vi "snake and ladders.vi"() -> ()   [LabVIEW 2018]
panel:
  out "?":bool
  out "x":dbl
  out "Number":dbl
  in  "ROLL":bool
  in  "stop":bool
  out "Ring":u16(ring)
  # "98"
  # "93"
  # "94"
  # "97"
  # "95"
  # "100"
  # "91"
  # "92"
  # "99"
  # "96"
  # "87"
  # "85"
  # "90"
  # "89"
  # "82"
  # "84"
  # "88"
  # "86"
  # "83"
  # "81"
  # "80"
  # "74"
  # "78"
  # "72"
  # "75"
  # "76"
  # "77"
  # "79"
  # "71"
  # "73"
  # "61"
  # "62"
  # "67"
  # "68"
  # "69"
  # "64"
  # "66"
  # "65"
  # "70"
  # "63"
  # "57"
  # "52"
  # "53"
  # "58"
  # "54"
  # "55"
  # "56"
  # "59"
  # "51"
  # "60"
  # "45"
  # "46"
  # "47"
  # "43"
  # "42"
  # "48"
  # "49"
  # "50"
  # "41"
  # "44"
  # "31"
  # "33"
  # "35"
  # "37"
  # "32"
  # "36"
  # "39"
  # "34"
  # "40"
  # "38"
  # "27"
  # "26"
  # "30"
  # "22"
  # "23"
  # "24"
  # "29"
  # "21"
  # "25"
  # "28"
  # "15"
  # "17"
  # "11"
  # "12"
  # "19"
  # "20"
  # "14"
  # "16"
  # "13"
  # "18"
  # "8"
  # "7"
  # "3"
  # "2"
  # "4"
  # "5"
  # "9"
  # "10"
  # "6"
  # "1"
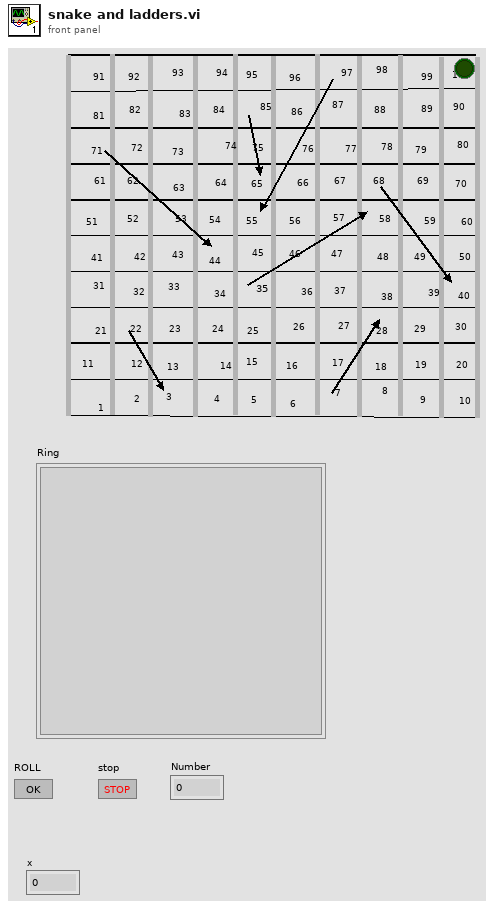
[diagram p1: front panel]
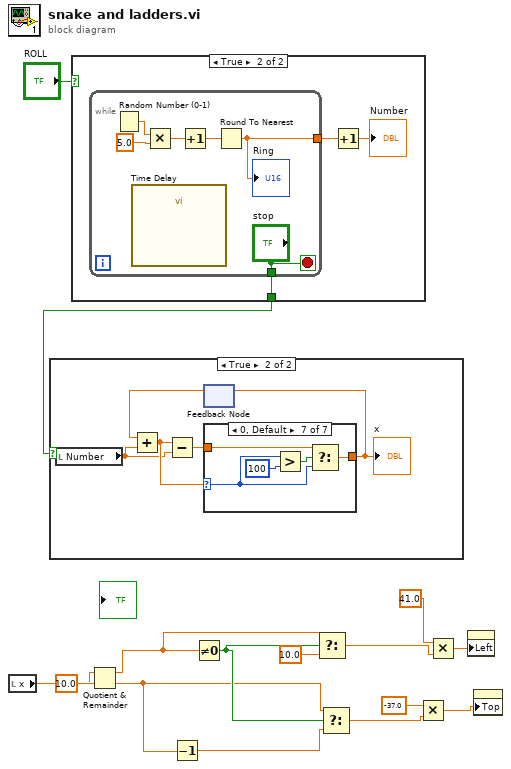
[diagram p0: block diagram]
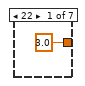
[diagram p3: hidden frame]
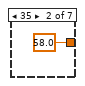
[diagram p4: hidden frame]
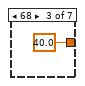
[diagram p5: hidden frame]
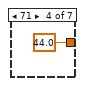
[diagram p6: hidden frame]
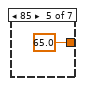
[diagram p7: hidden frame]
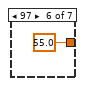
[diagram p8: hidden frame]
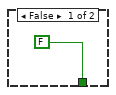
[diagram p9: hidden frame]
diagram:
  n1 = local read "x"() -> (w13:dbl)
  n2 = case shown="True" "ROLL" {
    tunnel: [FALSE ("Boolean") w17] -> w12
    frame False {
    }
    frame True {
      n3 = while {
        tunnel: [w21] -> w19
        tunnel: ["stop"] -> w17
        stop <- "stop" stop-if-true
        n4 = Random Number (0-1)() -> (number: 0 to 1=w25:dbl)
        n5 = call "Time Delay"() -> ()  [unwired: 11 in, 1 out]
        n6 = Multiply(x=w25, y=5.0) -> (x*y=w23:dbl)
        n7 = Increment(x=w23) -> (x+1=w22:dbl)
        n8 = Round To Nearest(number=w22) -> (nearest integer value=w21:dbl)
        "Ring" <- w21
      }
      n9 = Increment(x=w19) -> (x+1=→"Number":dbl)
    }
  }
  n10 = case shown="True" w12 {
    frame False {
    }
    frame True {
      n11 = local read "Number"() -> (w26:dbl)
      n12 = feedback #1() -> (w30:dbl)  [unwired: 1 in]
      n13 = Add(x=w30, y=w26) -> (x+y=w28:dbl)
      n14 = Subtract(x=w28, y=w26) -> (x-y=w27:dbl)
      n15 = case shown="0, Default" w28 {
        selector: w28 -> [_ _ _ _ _ _ w38]
        tunnel: [3.0 ("f") 58.0 ("f") 40.0 ("f") 44.0 ("f") 65.0 ("f") 55.0 ("f") w40] -> w29
        tunnel: w27 -> [_ _ _ _ _ _ w39]
        frame 22 {
        }
        frame 35 {
        }
        frame 68 {
        }
        frame 71 {
        }
        frame 85 {
        }
        frame 97 {
        }
        frame 0, Default {
          n16 = Greater?(x=w38, y=100 ("x")) -> (0:w41:bool)
          n17 = Select(t=w39, s=w41, f=w38) -> (s? t:f=w40:dbl)
        }
      }
      "x" <- w29
      n18 = feedback-in #1(w29) -> ()
    }
  }
  n19 = Quotient & Remainder(x=w13, y=10.0) -> (x-y*floor(x/y)=w9:dbl, floor(x/y)=w2:dbl)
  n20 = Decrement(x=w2) -> (x-1=w1:dbl)
  n21 = Not Equal To 0?(x=w9) -> (x != 0?=w4:bool)
  n22 = Select(t=w9, s=w4, f=10.0) -> (s? t:f=w7:dbl)
  n23 = Select(t=w2, s=w4, f=w1) -> (s? t:f=w3:dbl)
  n24 = Multiply(x=-37.0, y=w3) -> (x*y=w6:dbl)
  n25 = Multiply(x=41.0, y=w7) -> (x*y=w11:dbl)
  n26 = property class="Bool (strict)"("Left"=w11) -> ()  [unwired: 2 in, 2 out]
  n27 = property class="Bool (strict)"("Top"=w6) -> ()  [unwired: 2 in, 2 out]
